vi "Wait Time Step.vi"(5 "VolatusAPI":refnum<class "VolatusAPI.lvclass">, 6 "State Loop Data in":T1, 7 "State Control":T9, 9 "Seq Name":string, 11 "State in":refnum<class "State.lvclass">) -> (2 "Abort":bool, 3 "State out":refnum<class "State.lvclass">, 4 "State Loop Data":T1)   [LabVIEW 2023, in "VolatusSeq.lvlib" / "State.lvclass"]
uses:
  State.lvclass
  State Control.ctl
  Sequence Time.ctl
  Variables/Variables.lvclass
  State Loop Data.ctl
  Iteration Actions/Iteration Actions.lvclass
  Command.ctl
  Volatus/MessageQ/MessageQ.lvclass
  Format String/Format String.lvclass
  VolatusSeqConfig/Command Type.ctl
  messages/CmdDigital/Data.ctl
  messages/CmdAnalog/Data.ctl
  Send Type.ctl
  lv-vecto/Vecto/Channel DBL/Channel DBL.lvclass
  Transition/Transition.lvclass
  VolatusSeqConfig/Debug Flags.ctl
  State.lvclass/State.ctl
  Volatus/VolatusAPI/VolatusAPI.lvclass
  VolatusSeq.lvlib
  VolatusSeqConfig/VolatusSeqConfig.lvlib
  messages/CmdDigital/CmdDigital.lvlib
  messages/CmdAnalog/CmdAnalog.lvlib
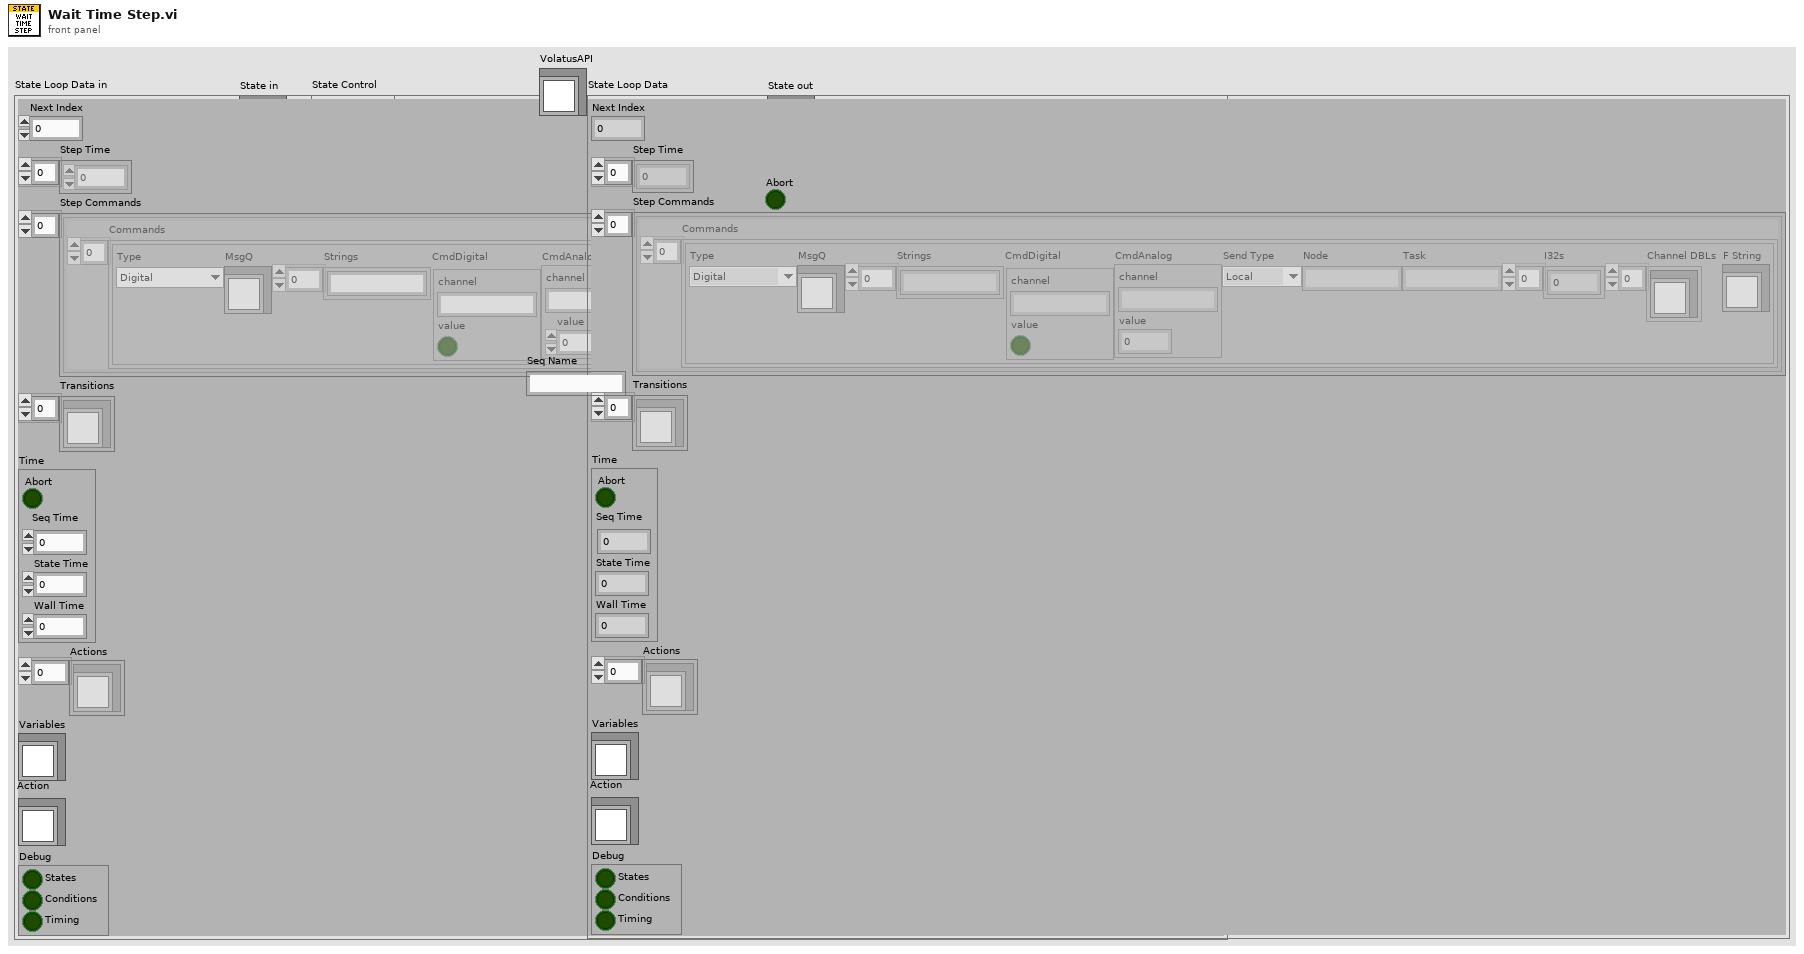
[diagram p1: front panel]
types:
  T1 = typedef "VolatusSeq.lvlib/State.lvclass/State Loop Data.ctl" = cluster{"Next Index":i32, "Step Time":dbl[], "Step Commands":cluster{"Commands":T2[]}[], "Transitions":refnum<class "Transition.lvclass">[], "Time":T7, "Actions":refnum<class "Iteration Actions.lvclass">[], "Variables":refnum<class "Variables.lvclass">, "Action":refnum<class "Iteration Actions.lvclass">, "Debug":T8}
  T2 = typedef "VolatusSeq.lvlib/Command.ctl" = cluster{"Type":T3, "MsgQ":refnum<class "MessageQ.lvclass">, "Strings":string[], "CmdDigital":T4, "CmdAnalog":T5, "Send Type":T6, "Node":string, "Task":string, "I32s":i32[], "Channel DBLs":refnum<class "Channel DBL.lvclass">[], "F String":refnum<class "Format String.lvclass">}
  T3 = typedef "VolatusSeqConfig.lvlib/Command Type.ctl" = enum16{"Digital", "Numeric", "Transition", "Stop", "StartLog", "StopLog", "Start", "Event", "Error", "HTTP", "ResetVar", "IncVar", "DecVar", "SaveVar", "LoadVar", "AddVar", "SubVar", "SetVar", "AddToVar"}
  T4 = typedef "CmdDigital.lvlib/Data.ctl" = cluster{"channel":string, "value":bool}
  T5 = typedef "CmdAnalog.lvlib/Data.ctl" = cluster{"channel":string, "value":dbl}
  T6 = typedef "VolatusSeq.lvlib/Send Type.ctl" = enum16{"Local", "Remote"}
  T7 = typedef "VolatusSeq.lvlib/Sequence Time.ctl" = cluster{"Abort":bool, "Seq Time":dbl, "State Time":dbl, "Wall Time":dbl}
  T8 = typedef "VolatusSeqConfig.lvlib/Debug Flags.ctl" = cluster{"States":bool, "Conditions":bool, "Timing":bool}
  T9 = typedef "VolatusSeq.lvlib/State Control.ctl" = cluster{"State":refnum<notifier>, "Time":refnum<notifier>, "Request State":refnum<notifier>, "Abort":refnum<notifier>, "Reset":refnum<notifier>, "Close":refnum<notifier>, "Vars SEQ":refnum<queue>}
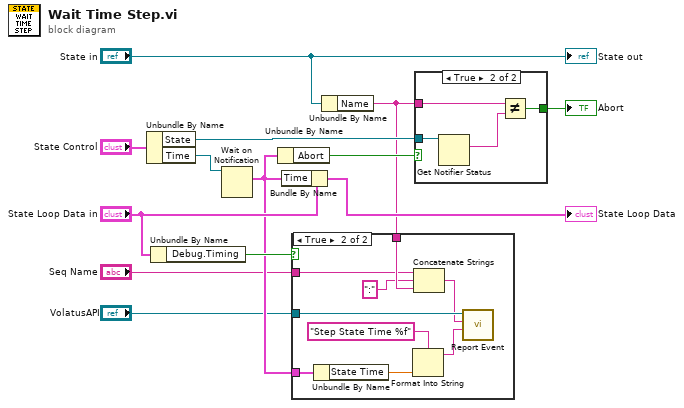
[diagram p0: block diagram]
diagram:
  n1 = Unbundle By Name("State Control") -> ("State"=w11:refnum<notifier>, "Time"=w12:refnum<notifier>)
  n2 = Unbundle By Name("State Loop Data in") -> ("Debug.Timing"=w5:bool)
  n3 = Wait on Notification(notifier=w12) -> (notification=w4:T7)  [unwired: 3 in, 3 out]
  n4 = Unbundle By Name(w4) -> ("Abort"=w10:bool)
  n5 = Bundle By Name(cluster="State Loop Data in", "Time"=w4) -> (→"State Loop Data":T1)
  n6 = Unbundle By Name("State in") -> ("Name"=w2:string)
  n7 = case shown="True" w5 {
    tunnel: w4 -> [_ w18]
    tunnel: "VolatusAPI" -> [_ w22]
    tunnel: w2 -> [_ w21]
    tunnel: "Seq Name" -> [_ w20]
    frame False {
    }
    frame True {
      n8 = Unbundle By Name(w18) -> ("State Time"=w17:dbl)
      n9 = Format Into String(format string="Step State Time %f", w17) -> (resulting string=w15:string)  [unwired: 2 in, 1 out]
      n10 = Concatenate Strings(w20, ":" ("string"), w21) -> (w19:string)
      n11 = call "Report Event.vi"("Message"=w15, "Context"=w19, "VolatusAPI in"=w22) -> ()  [unwired: 7 in, 2 out]
    }
  }
  n12 = case shown="True" w10 {
    tunnel: w11 -> [_ w26]
    tunnel: [_ w24] -> w7
    tunnel: w2 -> [_ w23]
    frame False {
    }
    frame True {
      n13 = Get Notifier Status(notifier=w26) -> (current notification=w25:string)  [unwired: 1 in, 4 out]
      n14 = Not Equal?(x=w23, y=w25) -> (x != y?=w24:bool)
    }
  }
  "Abort" <- w7
  "State out" <- "State in"
